vi "getGrating.vi"(8 "error in (no error)":errorcluster, 9 "Monochromator in":refnum<class "Monochromator.lvclass">, 11 "MonoState in":refnum<class "MonoState.lvclass">) -> (0 "error out":errorcluster, 1 "Monochromator out":refnum<class "Monochromator.lvclass">, 2 "GratingType":T1=enum."Red", 3 "MonoState out":refnum<class "MonoState.lvclass">)   [LabVIEW 2016, in "MonoState.lvclass"]
uses:
  MonoState.lvclass
  Typedefs/GratingType.ctl
  Monochromator/Monochromator.lvclass
  Monochromator/Monochromator.lvclass/Monochromator.ctl
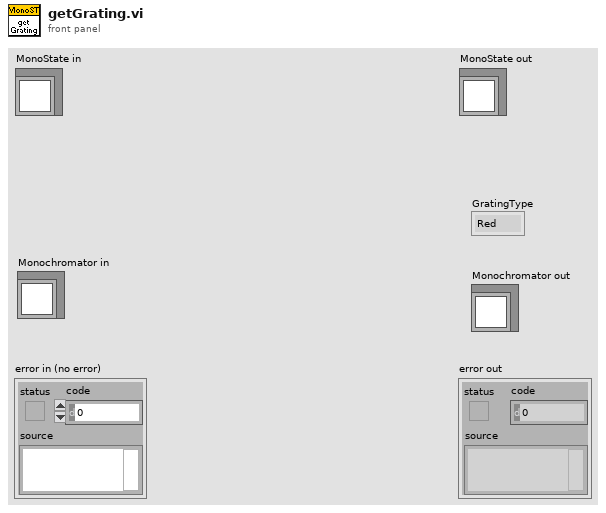
[diagram p1: front panel]
types:
  T1 = typedef "GratingType.ctl" = enum16{"Blue", "Red", "Mirror"}
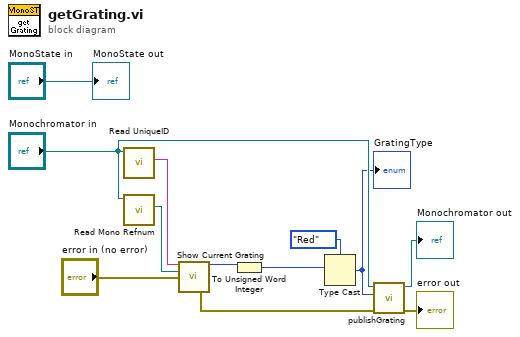
[diagram p0: block diagram]
diagram:
  n1 = call "Read UniqueID.vi"("Monochromator in"="Monochromator in") -> ("UniqueID"=w3:string)  [unwired: 8 in, 2 out]
  n2 = call "Read Mono Refnum.vi"("Monochromator in"="Monochromator in") -> ("Mono Refnum"=w4:refnum<k7>)  [unwired: 8 in, 2 out]
  n3 = call "Show Current Grating.vi"("UniqueID"=w3, "Refnum in"=w4, "error in (no error)"="error in (no error)") -> ("Grating Index"=w2:i32, "error out"=w6:errorcluster)  [unwired: 4 in, 7 out]
  n4 = To Unsigned Word Integer(number=w2) -> (unsigned 16bit integer=w1:u16)
  n5 = Type Cast(type=GratingType."Red" ("GratingType 2"), x=w1) -> (*(type *) &x=w7:T1)
  "GratingType" <- w7
  n6 = call "publishGrating.vi"("error in (no error)"=w6, "GratingType"=w7, "Monochromator in"="Monochromator in") -> ("error out"=→"error out":errorcluster, "Monochromator out"=→"Monochromator out":refnum<class "Monochromator.lvclass">)  [unwired: 7 in]
  "MonoState out" <- "MonoState in"
